vi "Cosine_distances.vi"(6 "Type Y":T2(ring), 7 "Type X":T2(ring), 8 "error in":errorcluster caption="entrée d'erreur", 10 "Y":string[][](array[string]), 11 "X":string[][](array[string])) -> (0 "error out":errorcluster caption="sortie d'erreur", 3 "Data":T1)   [LabVIEW 2020]
doc: "Compute cosine distance between samples in X and Y.\n\nCosine distance is defined as 1.0 minus the cosine similarity.\n\n\nParameters : \n\n- X : array_like, sparse matrix\nwith shape (n_samples_X, n_features).\n\n- Y : array_like, sparse matrix (optional)\nwith shape (n_samples_Y, n_features).\n\nReturns : \n\n- distance matrix : array\nAn array with shape (n_samples_X, n_samples_Y)."
uses:
  Cosine_distances.lvclass
panel:
  out "Cosine_distances.lvclass":refnum<class "Cosine_distances.lvclass">
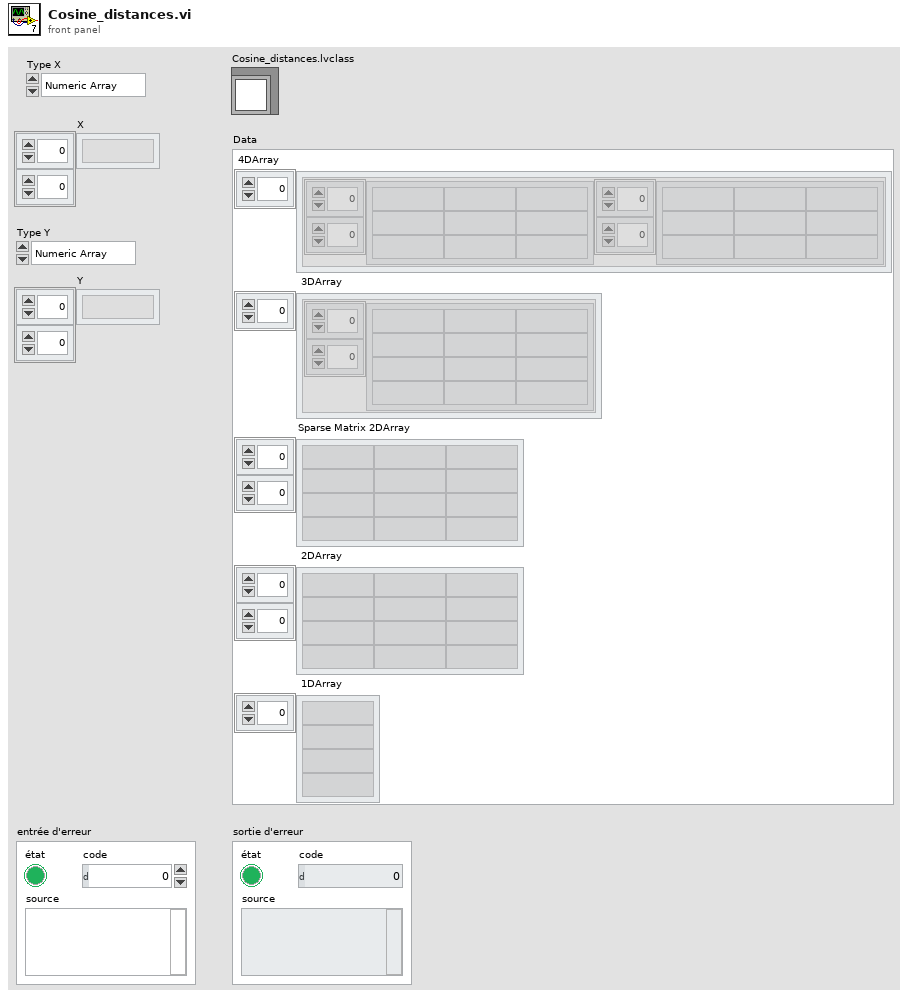
[diagram p1: front panel]
types:
  T1 = cluster{" 4DArray":cluster{"1":string[][], "2":string[][]}[], " 3DArray":cluster{"Tableau":string[][]}[], "Sparse Matrix 2DArray":string[][], " 2DArray":string[][], " 1DArray":string[]}
  T2 = enum16{"Numeric Array", "String Array", "Sparse"}
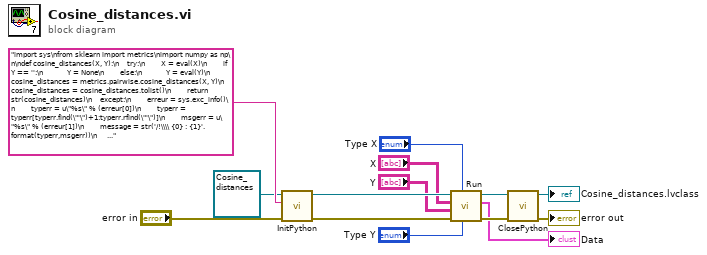
[diagram p0: block diagram]
diagram:
  n1 = call-dynamic "InitPython.vi"("error in (no error)"="error in", "Python Instruction"="import sys\nfrom sklearn import metrics\nimport numpy as np\n\ndef cosine_distances(X, Y):\n    try:\n        X = eval(X)\n        if Y == '':\n            Y = None\n        else:\n            Y = eval(Y)\n        cosine_distances = metrics.pairwise.cosine_distances(X, Y)\n        cosine_distances = cosine_distances.tolist()\n        return str(cosine_distances)\n    except:\n        erreur = sys.exc_info()\n        typerr = u\"%s\" % (erreur[0])\n        typerr = typerr[typerr.find(\"'\")+1:typerr.rfind(\"'\")]\n        msgerr = u\"%s\" % (erreur[1])\n        message = str('/!\\\\ {0} : {1}'. format(typerr,msgerr))\n        return message", "Scikit-learn en entrée"=refnum<class "Cosine_distances.lvclass"> refnum ("Cosine_distances.lvclass")) -> ("error out"=w11:errorcluster, "Scikit-learn en sortie"=w8:refnum<class "Cosine_distances.lvclass">)  [unwired: 7 in]
  n2 = call-dynamic "Run.vi"("Type Y"="Type Y", "Type X"="Type X", "error in (no error)"=w11, "Y"="Y", "X"="X", "Cosine_distances.lvclass"=w8) -> ("error out"=w10:errorcluster, "Data"=→"Data":T1, "Cosine_distances.lvclass"=w12:refnum<class "Cosine_distances.lvclass">)  [unwired: 3 in]
  n3 = call-dynamic "ClosePython.vi"("error in (no error)"=w10, "Scikit-learn en entrée"=w12) -> ("error out"=→"error out":errorcluster, "Scikit-learn en sortie"=→"Cosine_distances.lvclass":refnum<class "Cosine_distances.lvclass">)  [unwired: 8 in]
